vi "StatusAndPressure.vi"() -> ()   [LabVIEW 2019]
panel:
  out "Pressure 6":i32
  out "Status 6":string
  out "Pressure 5":i32
  out "Status 5":string
  out "Pressure 4":i32
  out "Status 4":string
  out "Pressure 3":i32
  out "Status 3":string
  out "Pressure 2":i32
  out "Status 2":string
  in  "stop":bool
  out "Pressure 1":i32
  out "Status 1":string
  out "Output 2":string
  in  "Delay":u32=500
  out "Output 1":string
  in  "VISA resource name":refnum<visa-resource-name>
  # "All pressures are displayed in mbar"
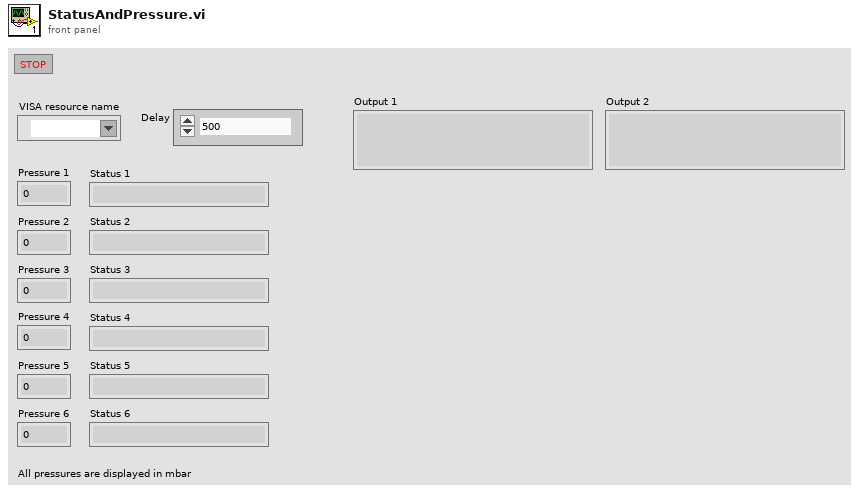
[diagram p1: front panel]
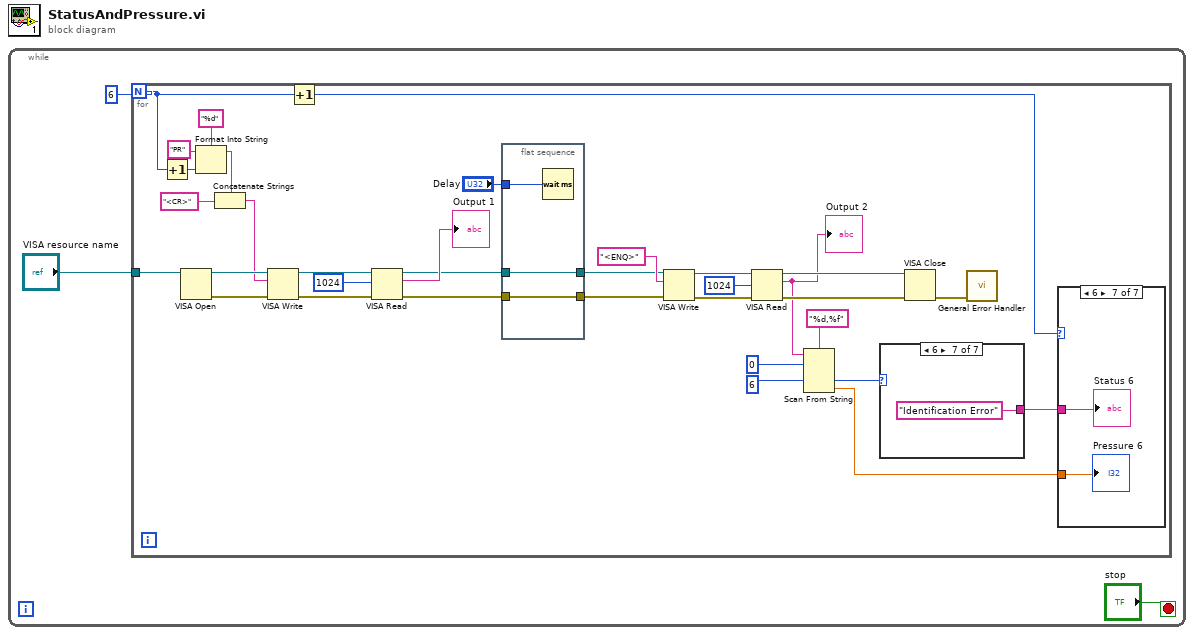
[diagram p0: block diagram]
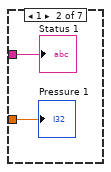
[diagram p3: hidden frame]
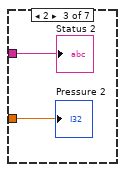
[diagram p4: hidden frame]
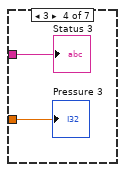
[diagram p5: hidden frame]
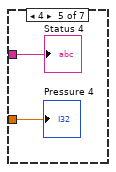
[diagram p6: hidden frame]
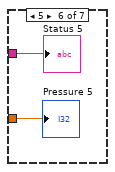
[diagram p7: hidden frame]
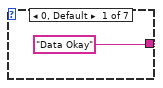
[diagram p8: hidden frame]
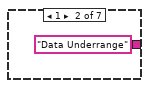
[diagram p9: hidden frame]
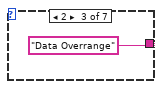
[diagram p10: hidden frame]
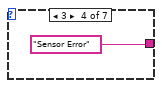
[diagram p11: hidden frame]
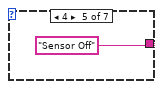
[diagram p12: hidden frame]
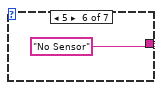
[diagram p13: hidden frame]
diagram:
  n1 = while {
    stop <- "stop" stop-if-true
    n2 = for {
      N: u32 6 ("unsigned 32bit integer") -> [w5]
      tunnel: "VISA resource name" -> [w24]
      n3 = Increment(x=w5) -> (x+1=w6:i32)
      n4 = VISA Open(VISA resource name=w24) -> (VISA resource name=w37:refnum<visa-resource-name>, error out=w35:errorcluster)  [unwired: 4 in]
      n5 = Format Into String(format string="%d", initial string="PR" ("String"), w6) -> (resulting string=w9:string)  [unwired: 1 in, 1 out]
      n6 = Concatenate Strings(w9, "<CR>" ("String")) -> (w7:string)
      n7 = VISA Write(VISA resource name=w37, write buffer=w7, error in (no error)=w35) -> (VISA resource name out=w36:refnum<visa-resource-name>, error out=w34:errorcluster)  [unwired: 1 out]
      n8 = Increment(x=w5) -> (x+1=w4:i32)
      n9 = VISA Read(VISA resource name=w36, byte count=u32 1024 ("unsigned 32bit integer"), error in (no error)=w34) -> (VISA resource name out=w22:refnum<visa-resource-name>, read buffer=→"Output 1":string, error out=w20:errorcluster)  [unwired: 1 out]
      n10 = flat-sequence {
        tunnel: "Delay" -> [w59]
        tunnel: [w58] -> w21
        tunnel: w22 -> [w58]
        tunnel: w20 -> [w57]
        tunnel: [w57] -> w19
        frame #0 {
          n11 = Wait (ms)(milliseconds to wait=w59) -> ()  [unwired: 1 out]
        }
      }
      n12 = VISA Write(VISA resource name=w21, write buffer="<ENQ>" ("String"), error in (no error)=w19) -> (VISA resource name out=w32:refnum<visa-resource-name>, error out=w30:errorcluster)  [unwired: 1 out]
      n13 = VISA Read(VISA resource name=w32, byte count=u32 1024 ("unsigned 32bit integer"), error in (no error)=w30) -> (VISA resource name out=w26:refnum<visa-resource-name>, read buffer=w18:string, error out=w28:errorcluster)  [unwired: 1 out]
      "Output 2" <- w18
      n14 = Scan From String(format string="%d,%f", input string=w18, initial scan location=u32 0 ("unsigned 32bit integer"), default 1=u32 6 ("unsigned 32bit integer")) -> (output 1=w15:u32, output 2=w13:dbl)  [unwired: 2 in, 3 out]
      n15 = case shown="6" w15 {
        tunnel: ["Data Okay" "Data Underrange" "Data Overrange" "Sensor Error" "Sensor Off" "No Sensor" "Identification Error"] -> w14
        frame 0, Default {
        }
        frame 1 {
        }
        frame 2 {
        }
        frame 3 {
        }
        frame 4 {
        }
        frame 5 {
        }
        frame 6 {
        }
      }
      n16 = VISA Close(VISA resource name=w26, error in (no error)=w28) -> (error out=w25:errorcluster)
      n17 = call <vilib>:"General Error Handler.vi"("error in (no error)"=w25) -> ()  [unwired: 10 in, 5 out]
      n18 = case shown="6" w4 {
        tunnel: w14 -> [_ w39 w41 w43 w45 w47 w49]
        tunnel: w13 -> [_ w38 w40 w42 w44 w46 w48]
        frame 0, Default {
        }
        frame 1 {
          "Status 1" <- w39
          "Pressure 1" <- w38
        }
        frame 2 {
          "Status 2" <- w41
          "Pressure 2" <- w40
        }
        frame 3 {
          "Status 3" <- w43
          "Pressure 3" <- w42
        }
        frame 4 {
          "Status 4" <- w45
          "Pressure 4" <- w44
        }
        frame 5 {
          "Status 5" <- w47
          "Pressure 5" <- w46
        }
        frame 6 {
          "Status 6" <- w49
          "Pressure 6" <- w48
        }
      }
    }
  }
